vi "UsrProfiles-Window-Profile name entry.vi"(6 "New user":bool, 7 "Colour":u32(colorbox)=16777225, 8 "error in (no error)":errorcluster, 11 "Profile name":string) -> (0 "error out":errorcluster, 1 "Cancelled (Left button pressed)":bool, 2 "New profile name":string)   [LabVIEW 2020]
doc: "Use this template to create a dialog box with event handling."
uses:
  <vilib>/Utility/miscctls.llb/LVPointTypeDef.ctl
  Global Variables/General Globals.vi
panel:
  in  "OK":bool
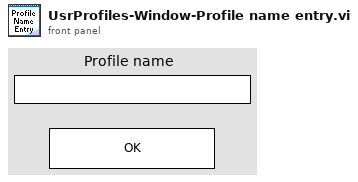
[diagram p1: front panel]
types:
  T1 = typedef "LVPointTypeDef.ctl" = cluster{"Horizontal":i16, "Vertical":i16}
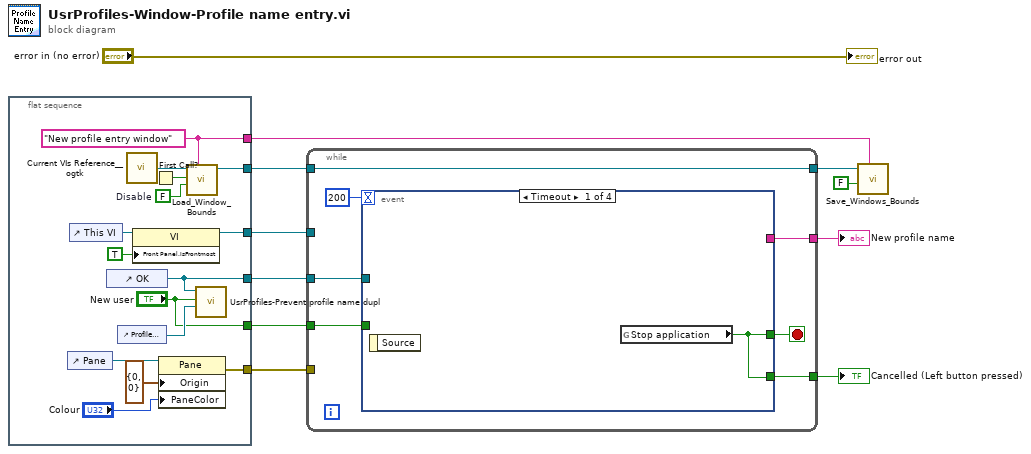
[diagram p0: block diagram]
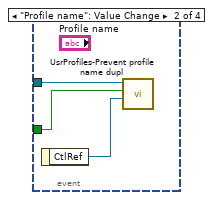
[diagram p2: hidden frame]
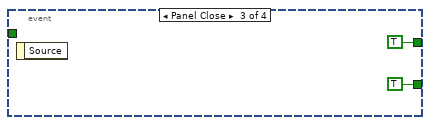
[diagram p3: hidden frame]
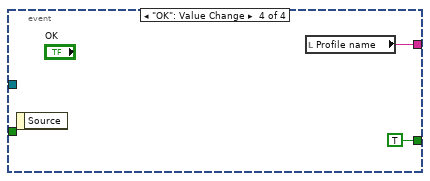
[diagram p4: hidden frame]
diagram:
  n1 = flat-sequence {
    tunnel: [w24] -> w11
    tunnel: [w22] -> w10
    tunnel: [w17] -> w8
    tunnel: [w16] -> w6
    tunnel: [w14] -> w2
    tunnel: ["New user"] -> w1
    frame #0 {
      w18 = FALSE  # Disable
      w17 = "New profile entry window" ("Window Name (i.e. Key)")
      n2 = control-ref of="Pane"() -> (w21:refnum<vi>)
      n3 = control-ref of="This VI"() -> (w25:refnum<vi>)
      n4 = control-ref of="OK"() -> (w14:refnum<vi>)
      n5 = control-ref of="Profile name"() -> (w13:refnum<vi>)
      n6 = call <userlib>:"Current VIs Reference__ogtk.vi"() -> ("Current VI's reference"=w20:refnum<vi>)  [unwired: 5 in]
      n7 = property on="Property Node" class="VI"(reference=w25, "Front Panel.IsFrontmost"=TRUE ("Front Panel Window:Is Frontmost")) -> (reference out=w24:refnum<vi>)  [unwired: 1 in, 1 out]
      n8 = First Call?() -> (First Call?: T/F=w19:bool)
      n9 = property class="Pane"(reference=w21, "Origin"=T1 {"Horizontal"=0, "Vertical"=0}, "PaneColor"="Colour") -> (error out=w22:errorcluster)  [unwired: 1 in, 1 out]
      n10 = call "Load_Window_Bounds.vi"("Window Name (i.e. Key)"=w17, "Disable"=w18, "First Call"=w19, "Window VI's Ref"=w20) -> ("reference out"=w16:refnum<vi>)  [unwired: 4 in, 3 out]
      n11 = call "UsrProfiles-Prevent profile name dupl.vi"("Profile name ref"=w13, "New user"="New user", "OK button ref"=w14) -> ()  [unwired: 9 in]
    }
  }
  n12 = while {
    tunnel: w10 -> [_]
    tunnel: w11 -> [_]
    tunnel: [w31] -> w9
    tunnel: w6 -> [w30]
    tunnel: [w30] -> w5
    tunnel: [w28] -> w3
    tunnel: w2 -> [w29]
    tunnel: w1 -> [w27]
    stop <- w33 stop-if-true
    n13 = event shown="[0] Timeout" {
      selector: _ -> [_ _ _ _]
      dyn-events: _ -> [_ _ _ _]
      timeout: 200 -> [_ _ _ _]
      tunnel: [w34 _ TRUE ("Stop?") TRUE ("Stop?")] -> w33
      tunnel: [w34 _ TRUE ("Stop subpanel") _] -> w31
      tunnel: w29 -> [_ w37 _ _]
      tunnel: [_ _ _ w40] -> w28
      tunnel: w27 -> [_ w36 _ _]
      event Timeout {
        n14 = event-data() -> ()  [unwired: 1 in, 1 out]
        n15 = global read "General Globals.vi" "Stop application"() -> (w34:bool)
      }
      event "Profile name": Value Change {
        n16 = event-data() -> ("CtlRef"=w35:refnum<vi>)  [unwired: 1 in]
        n17 = call "UsrProfiles-Prevent profile name dupl.vi"("Profile name ref"=w35, "New user"=w36, "OK button ref"=w37) -> ()  [unwired: 9 in]
      }
      event Panel Close {
        n18 = event-data() -> ()  [unwired: 1 in, 1 out]
      }
      event "OK": Value Change {
        n19 = event-data() -> ()  [unwired: 1 in, 1 out]
        n20 = local read "Profile name"() -> (w40:string)
      }
    }
  }
  "Cancelled (Left button pressed)" <- w9
  "New profile name" <- w3
  n21 = call "Save_Windows_Bounds.vi"("Window Name (i.e. Key)"=w8, "Front Panel Window:Open"=FALSE, "Window VI's Ref"=w5) -> ()  [unwired: 8 in, 1 out]
  "error out" <- "error in (no error)"
